vi "test-Coordinate-System-Test1.vi"() -> (3 "All tests passed":bool)   [LabVIEW 2019]
uses:
  <vilib>/Rock Robotics/WPI/ThirdParty/JAS_Junk/TrajLib/TypeDef/POSE3D.ctl
  <vilib>/Rock Robotics/WPI/ThirdParty/JAS_Junk/TrajLib/TypeDef/TRANSLATION3D.ctl
  <vilib>/Rock Robotics/WPI/ThirdParty/JAS_Junk/TrajLib/TypeDef/ROTATION3D.ctl
  <vilib>/Rock Robotics/WPI/ThirdParty/JAS_Junk/TrajLib/TypeDef/QUATERNION.ctl
  <vilib>/Rock Robotics/WPI/ThirdParty/JAS_Junk/TrajLib/VI/CoordAxis_N.vi
  <vilib>/Rock Robotics/WPI/ThirdParty/JAS_Junk/TrajLib/VI/CoordAxis_W.vi
  <vilib>/Rock Robotics/WPI/ThirdParty/JAS_Junk/TrajLib/VI/CoordAxis_U.vi
  <vilib>/Rock Robotics/WPI/ThirdParty/JAS_Junk/TrajLib/VI/CoordSystem_New.vi
  <vilib>/Rock Robotics/WPI/ThirdParty/JAS_Junk/TrajLib/VI/CoordAxis_E.vi
  <vilib>/Rock Robotics/WPI/ThirdParty/JAS_Junk/TrajLib/VI/CoordAxis_D.vi
  <vilib>/Rock Robotics/WPI/ThirdParty/JAS_Junk/TrajLib/Conv_Deg_Radians.vi
  <vilib>/Rock Robotics/WPI/ThirdParty/JAS_Junk/TrajLib/VI/Quaternion_New.vi
  <vilib>/Rock Robotics/WPI/ThirdParty/JAS_Junk/TrajLib/VI/Translation3d_Create.vi
  <vilib>/Rock Robotics/WPI/ThirdParty/JAS_Junk/TrajLib/VI/Pose3d_New_Trans3dRot3d.vi
  <vilib>/Rock Robotics/WPI/ThirdParty/JAS_Junk/TrajLib/VI/Rotation3d_Minus.vi
  <vilib>/Rock Robotics/WPI/ThirdParty/JAS_Junk/TrajLib/VI/Translation3d_Create_Default.vi
  <vilib>/Rock Robotics/WPI/ThirdParty/JAS_Junk/TrajLib/VI/Pose3d_RelativeTo.vi
  <vilib>/Rock Robotics/WPI/ThirdParty/JAS_Junk/TrajLib/VI/Rotation3d_RotateBy.vi
  <vilib>/Rock Robotics/WPI/ThirdParty/JAS_Junk/TrajLib/VI/Translation3d_RotateBy.vi
  <vilib>/Rock Robotics/WPI/ThirdParty/JAS_Junk/TrajLib/VI/Rotation3d_GetQuaterion.vi
  <vilib>/Rock Robotics/WPI/ThirdParty/JAS_Junk/TrajLib/VI/Quaternion_Equals.vi
  <vilib>/Rock Robotics/WPI/ThirdParty/JAS_Junk/TrajLib/VI/CoordAxis_New.vi
  <vilib>/Rock Robotics/WPI/ThirdParty/JAS_Junk/TrajLib/MatBuilder_Create.vi
  <vilib>/Rock Robotics/WPI/ThirdParty/JAS_Junk/TrajLib/Matrix_AssignBlock.vi
  <vilib>/Rock Robotics/WPI/ThirdParty/JAS_Junk/TrajLib/VI/Rotation3D_Create_RotMatrix.vi
  <vilib>/Rock Robotics/WPI/ThirdParty/JAS_Junk/TrajLib/VI/Rotation3d_UnaryMinus.vi
  <vilib>/Rock Robotics/WPI/ThirdParty/JAS_Junk/TrajLib/VI/Transform3d_Create_Pose3dPose3d.vi
  <vilib>/Rock Robotics/WPI/ThirdParty/JAS_Junk/TrajLib/VI/Transform3d_GetRotation3d.vi
  <vilib>/Rock Robotics/WPI/ThirdParty/JAS_Junk/TrajLib/VI/Transform3d_GetTranslation3d.vi
  <vilib>/Rock Robotics/WPI/ThirdParty/JAS_Junk/TrajLib/VI/Rotation3d_Create_Quaternion.vi
  <vilib>/Rock Robotics/WPI/ThirdParty/JAS_Junk/TrajLib/VI/Quaternion_Times.vi
  <vilib>/Rock Robotics/WPI/ThirdParty/JAS_Junk/TrajLib/VI/Quaternion_Inverse.vi
  <vilib>/Rock Robotics/WPI/ThirdParty/JAS_Junk/TrajLib/VI/Quaternion_Get_All.vi
  <vilib>/Rock Robotics/WPI/ThirdParty/JAS_Junk/TrajLib/VI/Quaternion_Get_Vect.vi
  <vilib>/Rock Robotics/WPI/ThirdParty/JAS_Junk/TrajLib/VI/Quaternion_Get_W.vi
  <vilib>/Rock Robotics/WPI/ThirdParty/JAS_Junk/TrajLib/MatrixHelper_CoerceSize.vi
  <vilib>/Rock Robotics/WPI/ThirdParty/JAS_Junk/TrajLib/Matrix_Transpose.vi
  <vilib>/Analysis/baseanly.llb/A x B.vi
  <vilib>/Analysis/baseanly.llb/Real A x B.vi
  <vilib>/Rock Robotics/WPI/ThirdParty/JAS_Junk/TrajLib/Matrix_Ident.vi
  <vilib>/Rock Robotics/WPI/ThirdParty/JAS_Junk/TrajLib/Matrix_IsEqual.vi
  <vilib>/Analysis/baseanly.llb/Determinant.vi
  <vilib>/Analysis/baseanly.llb/Real Determinant.vi
  <vilib>/Rock Robotics/WPI/ThirdParty/JAS_Junk/TrajLib/VI/Transform3d_Create_Trans3dRot3d.vi
  <vilib>/Rock Robotics/WPI/ThirdParty/JAS_Junk/TrajLib/VI/Translation3d_Minus.vi
  <vilib>/Rock Robotics/WPI/ThirdParty/JAS_Junk/TrajLib/VI/Quaternion_Normalize.vi
  <vilib>/Rock Robotics/WPI/ThirdParty/JAS_Junk/TrajLib/VI/Quaternion_New_Default.vi
  <vilib>/Analysis/Matrix/Numeric/Conversions/Array To Matrix.vi
  <vilib>/Analysis/Matrix/Numeric/Conversions/Array To Matrix - RA.vi
  <vilib>/Analysis/7linalg.llb/Create Special Matrix.vi
  <vilib>/Analysis/7linalg.llb/Create Special Real Matrix.vi
  <vilib>/Rock Robotics/WPI/ThirdParty/JAS_Junk/TrajLib/Trajectory_Library.lvlib
panel:
  out "out Pose3d":T1={"Translation3d"={"X"=0.0, "Y"=0.0, "Z"=0.0}, "Rotation3d"={"Q_quaternion"={"R"=1.0, "V"=[0.0, 0.0, 0.0]}}} {"Translation3d"."Z" format="%14.3f"; "Translation3d"."Y" format="%14.3f"; "Translation3d"."X" format="%14.3f"}
  out "out Converted Pose3d":T1={"Translation3d"={"X"=0.0, "Y"=0.0, "Z"=0.0}, "Rotation3d"={"Q_quaternion"={"R"=1.0, "V"=[0.0, 0.0, 0.0]}}} {"Translation3d"."Z" format="%14.3f"; "Translation3d"."Y" format="%14.3f"; "Translation3d"."X" format="%14.3f"}
  out "Test 4":bool
  out "Test 3":bool
  out "Test 2":bool
  out "Test 1":bool
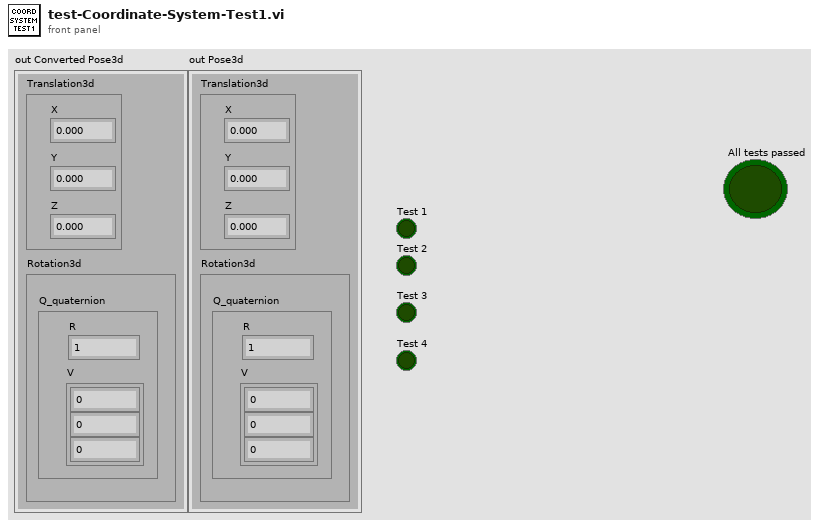
[diagram p1: front panel]
types:
  T1 = typedef "Trajectory_Library.lvlib/POSE3D.ctl" = cluster{"Translation3d":T2, "Rotation3d":T3}
  T2 = typedef "Trajectory_Library.lvlib/TRANSLATION3D.ctl" = cluster{"X":dbl, "Y":dbl, "Z":dbl}
  T3 = typedef "Trajectory_Library.lvlib/ROTATION3D.ctl" = cluster{"Q_quaternion":T4}
  T4 = typedef "Trajectory_Library.lvlib/QUATERNION.ctl" = cluster{"R":dbl, "V":dbl[]}
  T5 = typedef "Trajectory_Library.lvlib/COORDINATE_SYSTEM.ctl" = cluster{"Rotation":T3}
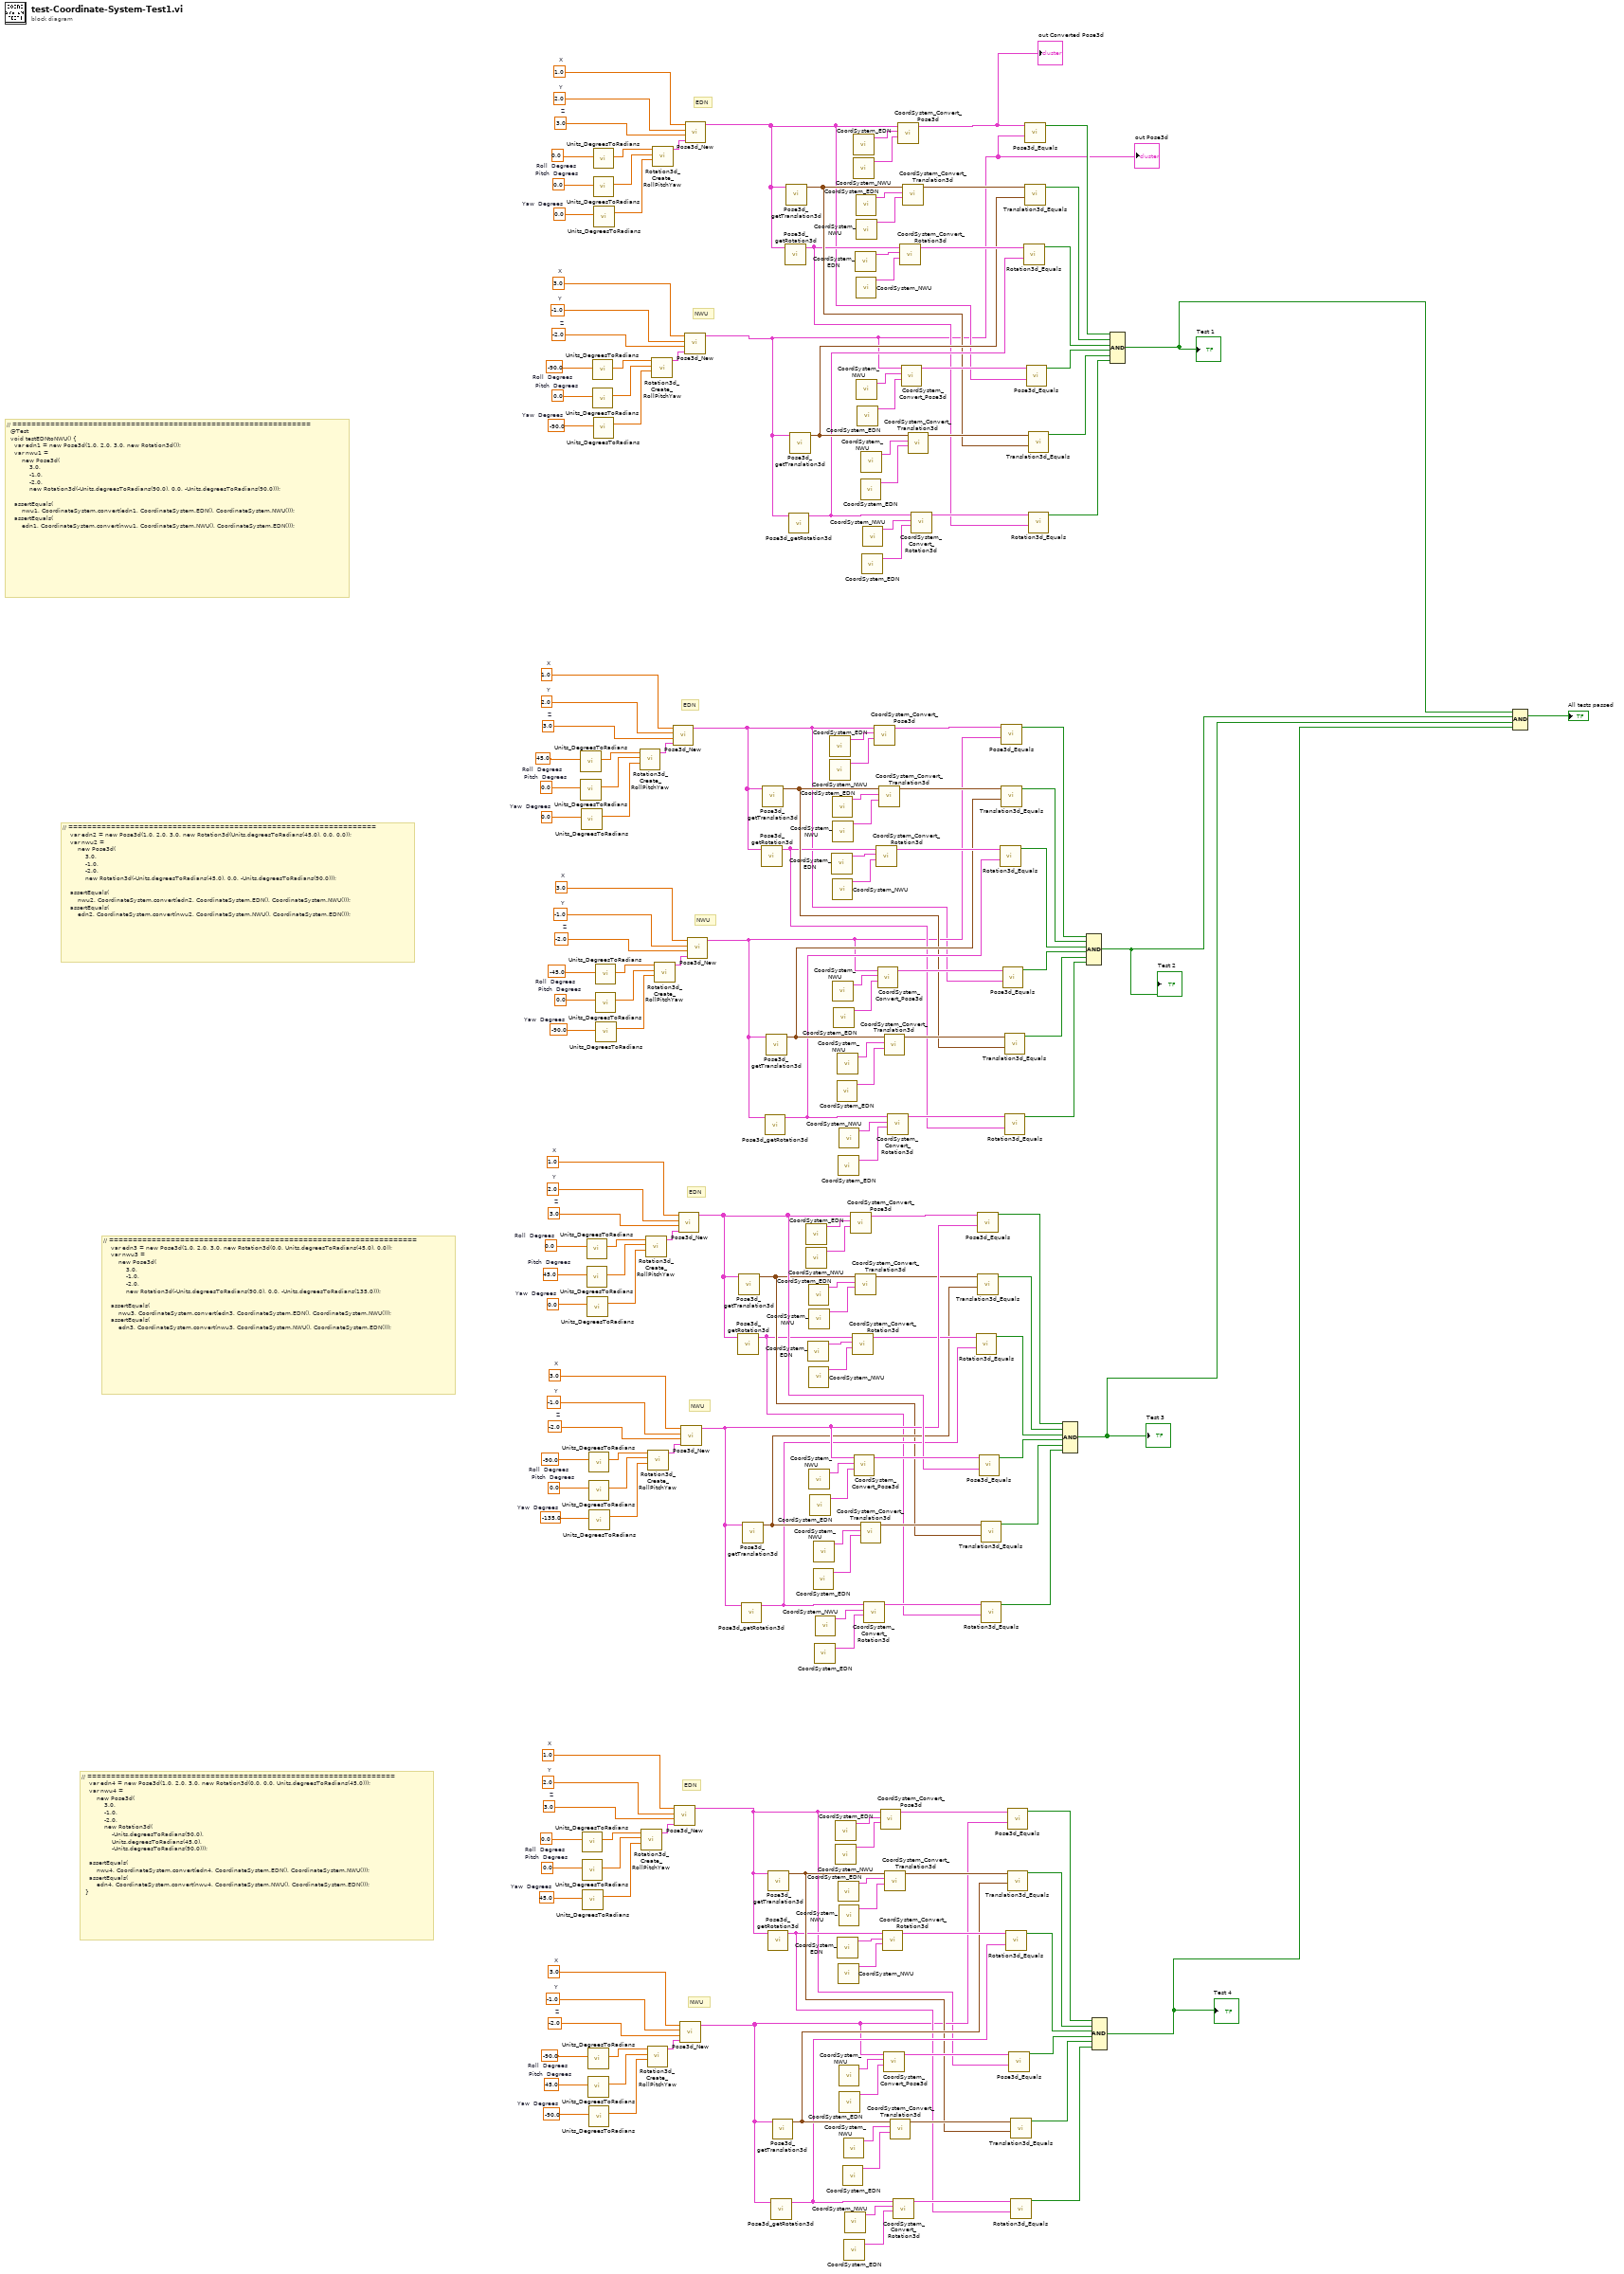
[diagram p0: block diagram]
diagram:
  w126 = 3.0  # X
  w125 = -1.0  # Y
  w124 = -2.0  # Z
  w118 = -90.0  # Roll  Degrees
  w119 = 45.0  # Pitch  Degrees
  w120 = -90.0  # Yaw  Degrees
  w136 = 1.0  # X
  w135 = 2.0  # Y
  w134 = 3.0  # Z
  w128 = 0.0  # Roll  Degrees
  w129 = 0.0  # Pitch  Degrees
  w130 = 45.0  # Yaw  Degrees
  w153 = 3.0  # X
  w152 = -1.0  # Y
  w151 = -2.0  # Z
  w145 = -90.0  # Roll  Degrees
  w146 = 0.0  # Pitch  Degrees
  w147 = -135.0  # Yaw  Degrees
  w163 = 1.0  # X
  w162 = 2.0  # Y
  w161 = 3.0  # Z
  w155 = 0.0  # Roll  Degrees
  w156 = 45.0  # Pitch  Degrees
  w157 = 0.0  # Yaw  Degrees
  w173 = 3.0  # X
  w172 = -1.0  # Y
  w171 = -2.0  # Z
  w165 = -45.0  # Roll  Degrees
  w166 = 0.0  # Pitch  Degrees
  w167 = -90.0  # Yaw  Degrees
  w183 = 1.0  # X
  w182 = 2.0  # Y
  w181 = 3.0  # Z
  w175 = 45.0  # Roll  Degrees
  w176 = 0.0  # Pitch  Degrees
  w177 = 0.0  # Yaw  Degrees
  w194 = 3.0  # X
  w193 = -1.0  # Y
  w192 = -2.0  # Z
  w186 = -90.0  # Roll  Degrees
  w187 = 0.0  # Pitch  Degrees
  w188 = -90.0  # Yaw  Degrees
  w204 = 1.0  # X
  w203 = 2.0  # Y
  w202 = 3.0  # Z
  w196 = 0.0  # Roll  Degrees
  w197 = 0.0  # Pitch  Degrees
  w198 = 0.0  # Yaw  Degrees
  # "// =================================================================\n    var edn2 = new Pose3d(1.0, 2.0, 3.0, new Rotation3d(Units.degreesToRadians(45.0), 0.0, 0.0));\n    var nwu2 =\n        new Pose3d(\n            3.0,\n            -1.0,\n            -2.0,\n            new Rotation3d(-Units.degreesToRadians(45.0), 0.0, -Units.degreesToRadians(90.0)));\n\n    assertEquals(\n        nwu2, CoordinateSystem.convert(edn2, CoordinateSystem.EDN(), CoordinateSystem.NWU()));\n    assertEquals(\n        edn2, CoordinateSystem.convert(nwu2, CoordinateSystem.NWU(), CoordinateSystem.EDN()));"
  # "// =================================================================\n    var edn3 = new Pose3d(1.0, 2.0, 3.0, new Rotation3d(0.0, Units.degreesToRadians(45.0), 0.0));\n    var nwu3 =\n        new Pose3d(\n            3.0,\n            -1.0,\n            -2.0,\n            new Rotation3d(-Units.degreesToRadians(90.0), 0.0, -Units.degreesToRadians(135.0)));\n\n    assertEquals(\n        nwu3, CoordinateSystem.convert(edn3, CoordinateSystem.EDN(), CoordinateSystem.NWU()));\n    assertEquals(\n        edn3, CoordinateSystem.convert(nwu3, CoordinateSystem.NWU(), CoordinateSystem.EDN()));"
  # "// =================================================================\n    var edn4 = new Pose3d(1.0, 2.0, 3.0, new Rotation3d(0.0, 0.0, Units.degreesToRadians(45.0)));\n    var nwu4 =\n        new Pose3d(\n            3.0,\n            -1.0,\n            -2.0,\n            new Rotation3d(\n                -Units.degreesToRadians(90.0),\n                Units.degreesToRadians(45.0),\n                -Units.degreesToRadians(90.0)));\n\n    assertEquals(\n        nwu4, CoordinateSystem.convert(edn4, CoordinateSystem.EDN(), CoordinateSystem.NWU()));\n    assertEquals(\n        edn4, CoordinateSystem.convert(nwu4, CoordinateSystem.NWU(), CoordinateSystem.EDN()));\n  }"
  # "NWU"
  # "EDN"
  # "NWU"
  # "EDN"
  # "NWU"
  # "EDN"
  # "NWU"
  # "EDN"
  # "// ===============================================================\n  @Test\n  void testEDNtoNWU() {\n    var edn1 = new Pose3d(1.0, 2.0, 3.0, new Rotation3d());\n    var nwu1 =\n        new Pose3d(\n            3.0,\n            -1.0,\n            -2.0,\n            new Rotation3d(-Units.degreesToRadians(90.0), 0.0, -Units.degreesToRadians(90.0)));\n\n    assertEquals(\n        nwu1, CoordinateSystem.convert(edn1, CoordinateSystem.EDN(), CoordinateSystem.NWU()));\n    assertEquals(\n        edn1, CoordinateSystem.convert(nwu1, CoordinateSystem.NWU(), CoordinateSystem.EDN()));"
  n1 = call <vilib>:"Units_DegreesToRadians.vi"("Degrees"=w175) -> ("Radians"=w178:dbl)  [unwired: 10 in]
  n2 = call <vilib>:"Units_DegreesToRadians.vi"("Degrees"=w176) -> ("Radians"=w179:dbl)  [unwired: 10 in]
  n3 = call <vilib>:"Units_DegreesToRadians.vi"("Degrees"=w177) -> ("Radians"=w180:dbl)  [unwired: 10 in]
  n4 = call <vilib>:"Units_DegreesToRadians.vi"("Degrees"=w128) -> ("Radians"=w131:dbl)  [unwired: 10 in]
  n5 = call <vilib>:"Units_DegreesToRadians.vi"("Degrees"=w129) -> ("Radians"=w132:dbl)  [unwired: 10 in]
  n6 = call <vilib>:"Units_DegreesToRadians.vi"("Degrees"=w130) -> ("Radians"=w133:dbl)  [unwired: 10 in]
  n7 = call <vilib>:"Units_DegreesToRadians.vi"("Degrees"=w155) -> ("Radians"=w158:dbl)  [unwired: 10 in]
  n8 = call <vilib>:"Units_DegreesToRadians.vi"("Degrees"=w156) -> ("Radians"=w159:dbl)  [unwired: 10 in]
  n9 = call <vilib>:"Units_DegreesToRadians.vi"("Degrees"=w157) -> ("Radians"=w160:dbl)  [unwired: 10 in]
  n10 = call <vilib>:"Units_DegreesToRadians.vi"("Degrees"=w118) -> ("Radians"=w121:dbl)  [unwired: 10 in]
  n11 = call <vilib>:"Units_DegreesToRadians.vi"("Degrees"=w119) -> ("Radians"=w122:dbl)  [unwired: 10 in]
  n12 = call <vilib>:"Units_DegreesToRadians.vi"("Degrees"=w145) -> ("Radians"=w148:dbl)  [unwired: 10 in]
  n13 = call <vilib>:"Units_DegreesToRadians.vi"("Degrees"=w146) -> ("Radians"=w149:dbl)  [unwired: 10 in]
  n14 = call <vilib>:"Units_DegreesToRadians.vi"("Degrees"=w120) -> ("Radians"=w123:dbl)  [unwired: 10 in]
  n15 = call <vilib>:"Units_DegreesToRadians.vi"("Degrees"=w147) -> ("Radians"=w150:dbl)  [unwired: 10 in]
  n16 = call <vilib>:"Units_DegreesToRadians.vi"("Degrees"=w186) -> ("Radians"=w189:dbl)  [unwired: 10 in]
  n17 = call <vilib>:"Units_DegreesToRadians.vi"("Degrees"=w187) -> ("Radians"=w190:dbl)  [unwired: 10 in]
  n18 = call <vilib>:"Units_DegreesToRadians.vi"("Degrees"=w196) -> ("Radians"=w199:dbl)  [unwired: 10 in]
  n19 = call <vilib>:"Units_DegreesToRadians.vi"("Degrees"=w197) -> ("Radians"=w200:dbl)  [unwired: 10 in]
  n20 = call <vilib>:"Units_DegreesToRadians.vi"("Degrees"=w188) -> ("Radians"=w191:dbl)  [unwired: 10 in]
  n21 = call <vilib>:"Units_DegreesToRadians.vi"("Degrees"=w198) -> ("Radians"=w201:dbl)  [unwired: 10 in]
  n22 = call <vilib>:"Units_DegreesToRadians.vi"("Degrees"=w165) -> ("Radians"=w168:dbl)  [unwired: 10 in]
  n23 = call <vilib>:"Units_DegreesToRadians.vi"("Degrees"=w166) -> ("Radians"=w169:dbl)  [unwired: 10 in]
  n24 = call <vilib>:"Units_DegreesToRadians.vi"("Degrees"=w167) -> ("Radians"=w170:dbl)  [unwired: 10 in]
  n25 = call <vilib>:"Rotation3d_Create_RollPitchYaw.vi"("Yaw"=w180, "Pitch"=w179, "Roll"=w178) -> ("Rotation3d"=w184:T3)  [unwired: 8 in]
  n26 = call <vilib>:"Rotation3d_Create_RollPitchYaw.vi"("Yaw"=w133, "Pitch"=w132, "Roll"=w131) -> ("Rotation3d"=w137:T3)  [unwired: 8 in]
  n27 = call <vilib>:"Rotation3d_Create_RollPitchYaw.vi"("Yaw"=w160, "Pitch"=w159, "Roll"=w158) -> ("Rotation3d"=w164:T3)  [unwired: 8 in]
  n28 = call <vilib>:"Rotation3d_Create_RollPitchYaw.vi"("Yaw"=w123, "Pitch"=w122, "Roll"=w121) -> ("Rotation3d"=w127:T3)  [unwired: 8 in]
  n29 = call <vilib>:"Rotation3d_Create_RollPitchYaw.vi"("Yaw"=w150, "Pitch"=w149, "Roll"=w148) -> ("Rotation3d"=w154:T3)  [unwired: 8 in]
  n30 = call <vilib>:"Rotation3d_Create_RollPitchYaw.vi"("Yaw"=w191, "Pitch"=w190, "Roll"=w189) -> ("Rotation3d"=w195:T3)  [unwired: 8 in]
  n31 = call <vilib>:"Rotation3d_Create_RollPitchYaw.vi"("Yaw"=w201, "Pitch"=w200, "Roll"=w199) -> ("Rotation3d"=w205:T3)  [unwired: 8 in]
  n32 = call <vilib>:"Rotation3d_Create_RollPitchYaw.vi"("Yaw"=w170, "Pitch"=w169, "Roll"=w168) -> ("Rotation3d"=w174:T3)  [unwired: 8 in]
  n33 = call <vilib>:"Pose3d_New.vi"("Rotation3d"=w184, "z"=w181, "Y"=w182, "X"=w183) -> ("out Pose3d"=w64:T1)  [unwired: 7 in]
  n34 = call <vilib>:"Pose3d_New.vi"("Rotation3d"=w137, "z"=w134, "Y"=w135, "X"=w136) -> ("out Pose3d"=w2:T1)  [unwired: 7 in]
  n35 = call <vilib>:"Pose3d_New.vi"("Rotation3d"=w164, "z"=w161, "Y"=w162, "X"=w163) -> ("out Pose3d"=w112:T1)  [unwired: 7 in]
  n36 = call <vilib>:"Pose3d_New.vi"("Rotation3d"=w127, "z"=w124, "Y"=w125, "X"=w126) -> ("out Pose3d"=w3:T1)  [unwired: 7 in]
  n37 = call <vilib>:"Pose3d_New.vi"("Rotation3d"=w154, "z"=w151, "Y"=w152, "X"=w153) -> ("out Pose3d"=w111:T1)  [unwired: 7 in]
  n38 = call <vilib>:"Pose3d_New.vi"("Rotation3d"=w195, "z"=w192, "Y"=w193, "X"=w194) -> ("out Pose3d"=w33:T1)  [unwired: 7 in]
  "out Pose3d" <- w33
  n39 = call <vilib>:"Pose3d_New.vi"("Rotation3d"=w205, "z"=w202, "Y"=w203, "X"=w204) -> ("out Pose3d"=w34:T1)  [unwired: 7 in]
  n40 = call <vilib>:"Pose3d_New.vi"("Rotation3d"=w174, "z"=w171, "Y"=w172, "X"=w173) -> ("out Pose3d"=w65:T1)  [unwired: 7 in]
  n41 = call <vilib>:"Pose3d_getRotation3d.vi"("in Pose3d"=w112) -> ("out Rotation3d"=w99:T3)  [unwired: 10 in]
  n42 = call <vilib>:"Pose3d_getTranslation3d.vi"("in Pose3d"=w112) -> ("out Translation3d"=w100:T2)  [unwired: 10 in]
  n43 = call <vilib>:"Pose3d_getRotation3d.vi"("in Pose3d"=w111) -> ("out Rotation3d"=w101:T3)  [unwired: 10 in]
  n44 = call <vilib>:"Pose3d_getTranslation3d.vi"("in Pose3d"=w111) -> ("out Translation3d"=w102:T2)  [unwired: 10 in]
  n45 = call <vilib>:"Pose3d_getRotation3d.vi"("in Pose3d"=w64) -> ("out Rotation3d"=w71:T3)  [unwired: 10 in]
  n46 = call <vilib>:"Pose3d_getTranslation3d.vi"("in Pose3d"=w64) -> ("out Translation3d"=w72:T2)  [unwired: 10 in]
  n47 = call <vilib>:"Pose3d_getRotation3d.vi"("in Pose3d"=w65) -> ("out Rotation3d"=w73:T3)  [unwired: 10 in]
  n48 = call <vilib>:"Pose3d_getTranslation3d.vi"("in Pose3d"=w65) -> ("out Translation3d"=w74:T2)  [unwired: 10 in]
  n49 = call <vilib>:"Pose3d_getRotation3d.vi"("in Pose3d"=w2) -> ("out Rotation3d"=w9:T3)  [unwired: 10 in]
  n50 = call <vilib>:"Pose3d_getTranslation3d.vi"("in Pose3d"=w2) -> ("out Translation3d"=w10:T2)  [unwired: 10 in]
  n51 = call <vilib>:"Pose3d_getRotation3d.vi"("in Pose3d"=w3) -> ("out Rotation3d"=w11:T3)  [unwired: 10 in]
  n52 = call <vilib>:"Pose3d_getTranslation3d.vi"("in Pose3d"=w3) -> ("out Translation3d"=w12:T2)  [unwired: 10 in]
  n53 = call <vilib>:"Pose3d_getRotation3d.vi"("in Pose3d"=w34) -> ("out Rotation3d"=w40:T3)  [unwired: 10 in]
  n54 = call <vilib>:"Pose3d_getTranslation3d.vi"("in Pose3d"=w34) -> ("out Translation3d"=w41:T2)  [unwired: 10 in]
  n55 = call <vilib>:"Pose3d_getRotation3d.vi"("in Pose3d"=w33) -> ("out Rotation3d"=w42:T3)  [unwired: 10 in]
  n56 = call <vilib>:"Pose3d_getTranslation3d.vi"("in Pose3d"=w33) -> ("out Translation3d"=w43:T2)  [unwired: 10 in]
  n57 = call <vilib>:"CoordSystem_EDN.vi"() -> ("out Coordinate System"=w144:T5)  [unwired: 10 in, 1 out]
  n58 = call <vilib>:"CoordSystem_NWU.vi"() -> ("out Coordinate System"=w143:T5)  [unwired: 10 in, 1 out]
  n59 = call <vilib>:"CoordSystem_EDN.vi"() -> ("out Coordinate System"=w114:T5)  [unwired: 10 in, 1 out]
  n60 = call <vilib>:"CoordSystem_EDN.vi"() -> ("out Coordinate System"=w116:T5)  [unwired: 10 in, 1 out]
  n61 = call <vilib>:"CoordSystem_NWU.vi"() -> ("out Coordinate System"=w113:T5)  [unwired: 10 in, 1 out]
  n62 = call <vilib>:"CoordSystem_NWU.vi"() -> ("out Coordinate System"=w115:T5)  [unwired: 10 in, 1 out]
  n63 = call <vilib>:"CoordSystem_NWU.vi"() -> ("out Coordinate System"=w142:T5)  [unwired: 10 in, 1 out]
  n64 = call <vilib>:"CoordSystem_EDN.vi"() -> ("out Coordinate System"=w141:T5)  [unwired: 10 in, 1 out]
  n65 = call <vilib>:"CoordSystem_EDN.vi"() -> ("out Coordinate System"=w109:T5)  [unwired: 10 in, 1 out]
  n66 = call <vilib>:"CoordSystem_NWU.vi"() -> ("out Coordinate System"=w110:T5)  [unwired: 10 in, 1 out]
  n67 = call <vilib>:"CoordSystem_EDN.vi"() -> ("out Coordinate System"=w107:T5)  [unwired: 10 in, 1 out]
  n68 = call <vilib>:"CoordSystem_NWU.vi"() -> ("out Coordinate System"=w108:T5)  [unwired: 10 in, 1 out]
  n69 = call <vilib>:"CoordSystem_EDN.vi"() -> ("out Coordinate System"=w93:T5)  [unwired: 10 in, 1 out]
  n70 = call <vilib>:"CoordSystem_NWU.vi"() -> ("out Coordinate System"=w92:T5)  [unwired: 10 in, 1 out]
  n71 = call <vilib>:"CoordSystem_EDN.vi"() -> ("out Coordinate System"=w84:T5)  [unwired: 10 in, 1 out]
  n72 = call <vilib>:"CoordSystem_EDN.vi"() -> ("out Coordinate System"=w86:T5)  [unwired: 10 in, 1 out]
  n73 = call <vilib>:"CoordSystem_NWU.vi"() -> ("out Coordinate System"=w83:T5)  [unwired: 10 in, 1 out]
  n74 = call <vilib>:"CoordSystem_NWU.vi"() -> ("out Coordinate System"=w85:T5)  [unwired: 10 in, 1 out]
  n75 = call <vilib>:"CoordSystem_NWU.vi"() -> ("out Coordinate System"=w91:T5)  [unwired: 10 in, 1 out]
  n76 = call <vilib>:"CoordSystem_EDN.vi"() -> ("out Coordinate System"=w90:T5)  [unwired: 10 in, 1 out]
  n77 = call <vilib>:"CoordSystem_EDN.vi"() -> ("out Coordinate System"=w31:T5)  [unwired: 10 in, 1 out]
  n78 = call <vilib>:"CoordSystem_NWU.vi"() -> ("out Coordinate System"=w30:T5)  [unwired: 10 in, 1 out]
  n79 = call <vilib>:"CoordSystem_EDN.vi"() -> ("out Coordinate System"=w81:T5)  [unwired: 10 in, 1 out]
  n80 = call <vilib>:"CoordSystem_NWU.vi"() -> ("out Coordinate System"=w82:T5)  [unwired: 10 in, 1 out]
  n81 = call <vilib>:"CoordSystem_EDN.vi"() -> ("out Coordinate System"=w22:T5)  [unwired: 10 in, 1 out]
  n82 = call <vilib>:"CoordSystem_EDN.vi"() -> ("out Coordinate System"=w79:T5)  [unwired: 10 in, 1 out]
  n83 = call <vilib>:"CoordSystem_EDN.vi"() -> ("out Coordinate System"=w24:T5)  [unwired: 10 in, 1 out]
  n84 = call <vilib>:"CoordSystem_NWU.vi"() -> ("out Coordinate System"=w21:T5)  [unwired: 10 in, 1 out]
  n85 = call <vilib>:"CoordSystem_NWU.vi"() -> ("out Coordinate System"=w80:T5)  [unwired: 10 in, 1 out]
  n86 = call <vilib>:"CoordSystem_NWU.vi"() -> ("out Coordinate System"=w23:T5)  [unwired: 10 in, 1 out]
  n87 = call <vilib>:"CoordSystem_NWU.vi"() -> ("out Coordinate System"=w29:T5)  [unwired: 10 in, 1 out]
  n88 = call <vilib>:"CoordSystem_EDN.vi"() -> ("out Coordinate System"=w28:T5)  [unwired: 10 in, 1 out]
  n89 = call <vilib>:"CoordSystem_EDN.vi"() -> ("out Coordinate System"=w19:T5)  [unwired: 10 in, 1 out]
  n90 = call <vilib>:"CoordSystem_NWU.vi"() -> ("out Coordinate System"=w20:T5)  [unwired: 10 in, 1 out]
  n91 = call <vilib>:"CoordSystem_EDN.vi"() -> ("out Coordinate System"=w17:T5)  [unwired: 10 in, 1 out]
  n92 = call <vilib>:"CoordSystem_NWU.vi"() -> ("out Coordinate System"=w18:T5)  [unwired: 10 in, 1 out]
  n93 = call <vilib>:"CoordSystem_Convert_Pose3d.vi"("CoordSys To"=w143, "CoordSys From"=w144, "in Pose3d"=w112) -> ("out Converted Pose3d"=w140:T1)  [unwired: 8 in]
  n94 = call <vilib>:"CoordSystem_Convert_Rotation3d.vi"("CoordSys To"=w113, "CoordSys From"=w114, "in Rotation3d"=w99) -> ("out Converted Rotation3d"=w105:T3)  [unwired: 8 in]
  n95 = call <vilib>:"CoordSystem_EDN.vi"() -> ("out Coordinate System"=w62:T5)  [unwired: 10 in, 1 out]
  n96 = call <vilib>:"CoordSystem_NWU.vi"() -> ("out Coordinate System"=w61:T5)  [unwired: 10 in, 1 out]
  n97 = call <vilib>:"CoordSystem_Convert_Pose3d.vi"("CoordSys To"=w141, "CoordSys From"=w142, "in Pose3d"=w111) -> ("out Converted Pose3d"=w139:T1)  [unwired: 8 in]
  n98 = call <vilib>:"CoordSystem_EDN.vi"() -> ("out Coordinate System"=w53:T5)  [unwired: 10 in, 1 out]
  n99 = call <vilib>:"CoordSystem_Convert_Translation3d.vi"("CoordSys To"=w115, "CoordSys From"=w116, "in Translation3d"=w100) -> ("out Converted Translation3d"=w106:T2)  [unwired: 8 in]
  n100 = call <vilib>:"CoordSystem_EDN.vi"() -> ("out Coordinate System"=w55:T5)  [unwired: 10 in, 1 out]
  n101 = call <vilib>:"CoordSystem_NWU.vi"() -> ("out Coordinate System"=w52:T5)  [unwired: 10 in, 1 out]
  n102 = call <vilib>:"CoordSystem_NWU.vi"() -> ("out Coordinate System"=w54:T5)  [unwired: 10 in, 1 out]
  n103 = call <vilib>:"CoordSystem_NWU.vi"() -> ("out Coordinate System"=w60:T5)  [unwired: 10 in, 1 out]
  n104 = call <vilib>:"CoordSystem_EDN.vi"() -> ("out Coordinate System"=w59:T5)  [unwired: 10 in, 1 out]
  n105 = call <vilib>:"CoordSystem_EDN.vi"() -> ("out Coordinate System"=w50:T5)  [unwired: 10 in, 1 out]
  n106 = call <vilib>:"CoordSystem_Convert_Translation3d.vi"("CoordSys To"=w109, "CoordSys From"=w110, "in Translation3d"=w102) -> ("out Converted Translation3d"=w104:T2)  [unwired: 8 in]
  n107 = call <vilib>:"CoordSystem_NWU.vi"() -> ("out Coordinate System"=w51:T5)  [unwired: 10 in, 1 out]
  n108 = call <vilib>:"CoordSystem_EDN.vi"() -> ("out Coordinate System"=w48:T5)  [unwired: 10 in, 1 out]
  n109 = call <vilib>:"CoordSystem_NWU.vi"() -> ("out Coordinate System"=w49:T5)  [unwired: 10 in, 1 out]
  n110 = call <vilib>:"CoordSystem_Convert_Rotation3d.vi"("CoordSys To"=w107, "CoordSys From"=w108, "in Rotation3d"=w101) -> ("out Converted Rotation3d"=w103:T3)  [unwired: 8 in]
  n111 = call <vilib>:"CoordSystem_Convert_Pose3d.vi"("CoordSys To"=w92, "CoordSys From"=w93, "in Pose3d"=w64) -> ("out Converted Pose3d"=w89:T1)  [unwired: 8 in]
  n112 = call <vilib>:"CoordSystem_Convert_Rotation3d.vi"("CoordSys To"=w83, "CoordSys From"=w84, "in Rotation3d"=w71) -> ("out Converted Rotation3d"=w77:T3)  [unwired: 8 in]
  n113 = call <vilib>:"CoordSystem_Convert_Pose3d.vi"("CoordSys To"=w90, "CoordSys From"=w91, "in Pose3d"=w65) -> ("out Converted Pose3d"=w88:T1)  [unwired: 8 in]
  n114 = call <vilib>:"CoordSystem_Convert_Translation3d.vi"("CoordSys To"=w85, "CoordSys From"=w86, "in Translation3d"=w72) -> ("out Converted Translation3d"=w78:T2)  [unwired: 8 in]
  n115 = call <vilib>:"CoordSystem_Convert_Pose3d.vi"("CoordSys To"=w30, "CoordSys From"=w31, "in Pose3d"=w2) -> ("out Converted Pose3d"=w27:T1)  [unwired: 8 in]
  n116 = call <vilib>:"CoordSystem_Convert_Rotation3d.vi"("CoordSys To"=w21, "CoordSys From"=w22, "in Rotation3d"=w9) -> ("out Converted Rotation3d"=w15:T3)  [unwired: 8 in]
  n117 = call <vilib>:"CoordSystem_Convert_Pose3d.vi"("CoordSys To"=w28, "CoordSys From"=w29, "in Pose3d"=w3) -> ("out Converted Pose3d"=w26:T1)  [unwired: 8 in]
  n118 = call <vilib>:"CoordSystem_Convert_Translation3d.vi"("CoordSys To"=w81, "CoordSys From"=w82, "in Translation3d"=w74) -> ("out Converted Translation3d"=w76:T2)  [unwired: 8 in]
  n119 = call <vilib>:"CoordSystem_Convert_Translation3d.vi"("CoordSys To"=w23, "CoordSys From"=w24, "in Translation3d"=w10) -> ("out Converted Translation3d"=w16:T2)  [unwired: 8 in]
  n120 = call <vilib>:"CoordSystem_Convert_Rotation3d.vi"("CoordSys To"=w79, "CoordSys From"=w80, "in Rotation3d"=w73) -> ("out Converted Rotation3d"=w75:T3)  [unwired: 8 in]
  n121 = call <vilib>:"CoordSystem_Convert_Translation3d.vi"("CoordSys To"=w19, "CoordSys From"=w20, "in Translation3d"=w12) -> ("out Converted Translation3d"=w14:T2)  [unwired: 8 in]
  n122 = call <vilib>:"CoordSystem_Convert_Rotation3d.vi"("CoordSys To"=w17, "CoordSys From"=w18, "in Rotation3d"=w11) -> ("out Converted Rotation3d"=w13:T3)  [unwired: 8 in]
  n123 = call <vilib>:"CoordSystem_Convert_Pose3d.vi"("CoordSys To"=w61, "CoordSys From"=w62, "in Pose3d"=w34) -> ("out Converted Pose3d"=w58:T1)  [unwired: 8 in]
  "out Converted Pose3d" <- w58
  n124 = call <vilib>:"CoordSystem_Convert_Rotation3d.vi"("CoordSys To"=w52, "CoordSys From"=w53, "in Rotation3d"=w40) -> ("out Converted Rotation3d"=w46:T3)  [unwired: 8 in]
  n125 = call <vilib>:"CoordSystem_Convert_Pose3d.vi"("CoordSys To"=w59, "CoordSys From"=w60, "in Pose3d"=w33) -> ("out Converted Pose3d"=w57:T1)  [unwired: 8 in]
  n126 = call <vilib>:"CoordSystem_Convert_Translation3d.vi"("CoordSys To"=w54, "CoordSys From"=w55, "in Translation3d"=w41) -> ("out Converted Translation3d"=w47:T2)  [unwired: 8 in]
  n127 = call <vilib>:"CoordSystem_Convert_Translation3d.vi"("CoordSys To"=w50, "CoordSys From"=w51, "in Translation3d"=w43) -> ("out Converted Translation3d"=w45:T2)  [unwired: 8 in]
  n128 = call <vilib>:"CoordSystem_Convert_Rotation3d.vi"("CoordSys To"=w48, "CoordSys From"=w49, "in Rotation3d"=w42) -> ("out Converted Rotation3d"=w44:T3)  [unwired: 8 in]
  n129 = call <vilib>:"Rotation3d_Equals.vi"("other Rotation3d"=w101, "in Rotation3d"=w105) -> ("Equals"=w94:bool)  [unwired: 9 in]
  n130 = call <vilib>:"Pose3d_Equals.vi"("other Pose3d"=w111, "in Pose3d"=w140) -> ("Equals"=w96:bool)  [unwired: 9 in]
  n131 = call <vilib>:"Translation3d_Equals.vi"("other Translation3d"=w102, "In Translation3d"=w106) -> ("Equals"=w95:bool)  [unwired: 9 in]
  n132 = call <vilib>:"Pose3d_Equals.vi"("other Pose3d"=w112, "in Pose3d"=w139) -> ("Equals"=w138:bool)  [unwired: 9 in]
  n133 = call <vilib>:"Translation3d_Equals.vi"("other Translation3d"=w100, "In Translation3d"=w104) -> ("Equals"=w98:bool)  [unwired: 9 in]
  n134 = call <vilib>:"Rotation3d_Equals.vi"("other Rotation3d"=w99, "in Rotation3d"=w103) -> ("Equals"=w97:bool)  [unwired: 9 in]
  n135 = call <vilib>:"Rotation3d_Equals.vi"("other Rotation3d"=w73, "in Rotation3d"=w77) -> ("Equals"=w66:bool)  [unwired: 9 in]
  n136 = call <vilib>:"Pose3d_Equals.vi"("other Pose3d"=w65, "in Pose3d"=w89) -> ("Equals"=w68:bool)  [unwired: 9 in]
  n137 = call <vilib>:"Translation3d_Equals.vi"("other Translation3d"=w74, "In Translation3d"=w78) -> ("Equals"=w67:bool)  [unwired: 9 in]
  n138 = call <vilib>:"Pose3d_Equals.vi"("other Pose3d"=w64, "in Pose3d"=w88) -> ("Equals"=w87:bool)  [unwired: 9 in]
  n139 = call <vilib>:"Translation3d_Equals.vi"("other Translation3d"=w72, "In Translation3d"=w76) -> ("Equals"=w70:bool)  [unwired: 9 in]
  n140 = call <vilib>:"Rotation3d_Equals.vi"("other Rotation3d"=w71, "in Rotation3d"=w75) -> ("Equals"=w69:bool)  [unwired: 9 in]
  n141 = call <vilib>:"Rotation3d_Equals.vi"("other Rotation3d"=w11, "in Rotation3d"=w15) -> ("Equals"=w4:bool)  [unwired: 9 in]
  n142 = call <vilib>:"Pose3d_Equals.vi"("other Pose3d"=w3, "in Pose3d"=w27) -> ("Equals"=w6:bool)  [unwired: 9 in]
  n143 = call <vilib>:"Translation3d_Equals.vi"("other Translation3d"=w12, "In Translation3d"=w16) -> ("Equals"=w5:bool)  [unwired: 9 in]
  n144 = call <vilib>:"Pose3d_Equals.vi"("other Pose3d"=w2, "in Pose3d"=w26) -> ("Equals"=w25:bool)  [unwired: 9 in]
  n145 = call <vilib>:"Translation3d_Equals.vi"("other Translation3d"=w10, "In Translation3d"=w14) -> ("Equals"=w8:bool)  [unwired: 9 in]
  n146 = call <vilib>:"Rotation3d_Equals.vi"("other Rotation3d"=w9, "in Rotation3d"=w13) -> ("Equals"=w7:bool)  [unwired: 9 in]
  n147 = call <vilib>:"Rotation3d_Equals.vi"("other Rotation3d"=w42, "in Rotation3d"=w46) -> ("Equals"=w35:bool)  [unwired: 9 in]
  n148 = call <vilib>:"Pose3d_Equals.vi"("other Pose3d"=w33, "in Pose3d"=w58) -> ("Equals"=w37:bool)  [unwired: 9 in]
  n149 = call <vilib>:"Translation3d_Equals.vi"("other Translation3d"=w43, "In Translation3d"=w47) -> ("Equals"=w36:bool)  [unwired: 9 in]
  n150 = call <vilib>:"Pose3d_Equals.vi"("other Pose3d"=w34, "in Pose3d"=w57) -> ("Equals"=w56:bool)  [unwired: 9 in]
  n151 = call <vilib>:"Translation3d_Equals.vi"("other Translation3d"=w41, "In Translation3d"=w45) -> ("Equals"=w39:bool)  [unwired: 9 in]
  n152 = call <vilib>:"Rotation3d_Equals.vi"("other Rotation3d"=w40, "in Rotation3d"=w44) -> ("Equals"=w38:bool)  [unwired: 9 in]
  n153 = Compound Arithmetic op=AND(w96, w95, w94, w138, w98, w97) -> (w117:bool)
  "Test 3" <- w117
  n154 = Compound Arithmetic op=AND(w68, w67, w66, w87, w70, w69) -> (w63:bool)
  "Test 2" <- w63
  n155 = Compound Arithmetic op=AND(w6, w5, w4, w25, w8, w7) -> (w1:bool)
  "Test 4" <- w1
  n156 = Compound Arithmetic op=AND(w37, w36, w35, w56, w39, w38) -> (w32:bool)
  "Test 1" <- w32
  n157 = Compound Arithmetic op=AND(w32, w63, w117, w1) -> (→"All tests passed":bool)
